vi "finalDOchannelselecthack.vi"() -> (1 "usedDO":u32[](array[numeric]), 2 "presorted indices":u32[](array[numeric]))   [LabVIEW 2015]
uses:
  Objects/configuration.vi
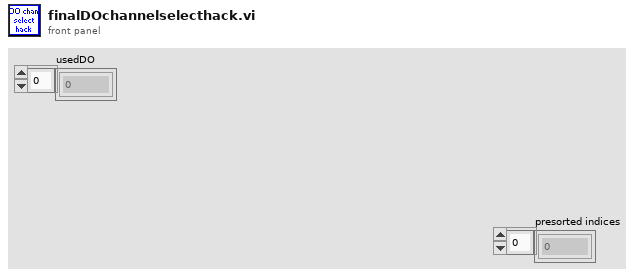
[diagram p1: front panel]
types:
  T1 = typedef "LVRectTypeDef.ctl" = cluster{"Left":i16, "Top":i16, "Right":i16, "Bottom":i16}
  T2 = cluster{"Xpixels":i32, "Vxminref":dbl, "Vxmaxref":dbl, "P":dbl, "Ypixels":i32, "Vyminref":dbl, "Vymaxref":dbl, "srate":sgl, "sAOxy":i32, "timeout":dbl, "type":string, "date":string, "time":string, "Colormap":u16, "Drawing Mode":u16, "Scanning Mode":u16, "square pixels":bool, "square matrix":bool, "Xpixels Img":i32, "Vx-min Img":dbl, "VX-max Img":dbl, "Ypixels Img":i32, "Vy-min Img":dbl, "Vy-max Img ":dbl, "Angle Img":dbl, "autoshutter":bool, "finite":bool, "cont":bool, "wavdet":bool, "measpoints":i32, "avpp":i32, "bufferAO":i32, "bufferAI":i32, "starttick":u32, "waveform":path, "Vx-ref":dbl, "Vy-ref":dbl, "refreshrate":dbl, "refreshbuffer":i32, "tt_cycles":i32, "motorref":refnum<k7>, "mirrorswitch":refnum<k7>, "sample mode":i32, "maxbufferAI":i32, "srateAODO":sgl, "bin":sgl, "Pel":sgl, "Angle draw":dbl, "srate Img":sgl, "ROIimg_plotbounds":T1, "auto OD":bool, "ODfilt":u16, "aAI":i32[], "aCI":i32[], "aAO":u32[], "aDO":u32[], "refwfsize":dbl, "Lifetime":bool, "Vz-Img":dbl, "Vz-ref":dbl, "Vz-reset":dbl, "AIoverride":bool}
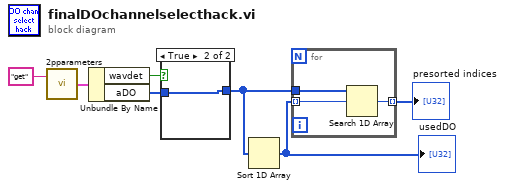
[diagram p0: block diagram]
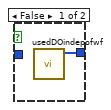
[diagram p2: hidden frame]
diagram:
  n1 = call "2pparameters.vi"("command"="get") -> ("params out"=w6:T2)  [unwired: 1 in]
  n2 = Unbundle By Name(w6) -> ("wavdet"=w4:bool, "aDO"=w5:u32[])
  n3 = case shown="True" w4 {
    tunnel: w5 -> [_ w9]
    tunnel: [w8 w9] -> w2
    frame False {
      n4 = call "usedDOindepofwf.vi"() -> ("DO"=w8:u32[])  [unwired: 11 in]
    }
    frame True {
    }
  }
  n5 = Sort 1D Array(array=w2) -> (sorted array=w1:u32[])
  "usedDO" <- w1
  n6 = for {
    tunnel: w1 -> [w12] mode=indexing
    tunnel: w2 -> [w11]
    tunnel: [w10] -> w3 mode=indexing
    n7 = Search 1D Array(1D array=w11, element=w12) -> (index of element=w10:i32)  [unwired: 1 in]
  }
  "presorted indices" <- w3
